vi "Open serial.vi"(8 "error in (no error)":errorcluster, 10 "port":string, 11 "SIM_Roda_Filtros in":refnum<class "SIM_Roda_Filtros.lvclass">) -> (0 "error out":errorcluster, 2 "status":bool, 3 "SIM_Roda_Filtros out":refnum<class "SIM_Roda_Filtros.lvclass">)   [LabVIEW 2018, in "SIM_Roda_Filtros.lvclass"]
uses:
  SIM_Roda_Filtros.lvclass
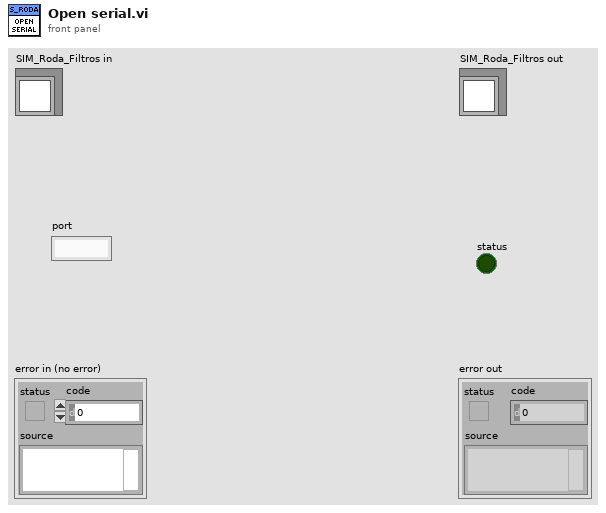
[diagram p1: front panel]
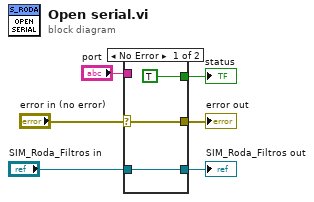
[diagram p0: block diagram]
diagram:
  n1 = case shown="No Error" "error in (no error)" {
    selector: "error in (no error)" -> [w9 w10]
    tunnel: [w9 w10] -> w5
    tunnel: "port" -> [_ _]
    tunnel: "SIM_Roda_Filtros in" -> [w8 w11]
    tunnel: [w8 w11] -> w2
    tunnel: [TRUE _] -> w1
    frame No Error {
    }
    frame Error {
    }
  }
  "error out" <- w5
  "SIM_Roda_Filtros out" <- w2
  "status" <- w1
